vi "Convert LIN Trace to Raw Frame.vi"(8 "error in":errorcluster, 11 "captured data in":string[][](array[string])) -> (0 "error out":errorcluster, 2 "raw frames":u8[](array[numeric]) format="%02x")   [LabVIEW 2025, in "CAN-LIN Raw Bus Capture UI.lvlib"]
uses:
  CAN-LIN Raw Bus Capture UI.lvlib
  <vilib>/xnet/xnet.llb/XNET Frame Type LIN.ctl
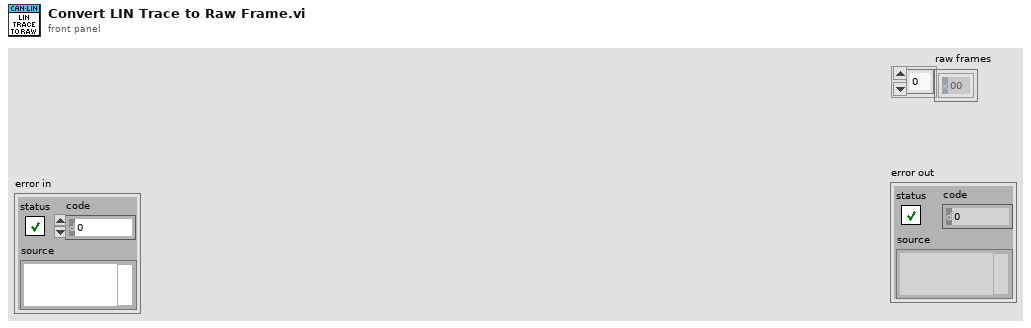
[diagram p1: front panel]
types:
  T1 = typedef "XNET Frame Type LIN.ctl" = u8
  T2 = cluster{"timestamp":timestamp, "payload":u8[], "identifier":u32, "type":T1, "event ID":u8, "event slot?":bool, "echo?":bool}[]
  T3 = cluster{"timestamp":timestamp, "payload":u8[], "identifier":u32, "type":T1, "event ID":u8, "event slot?":bool, "echo?":bool}
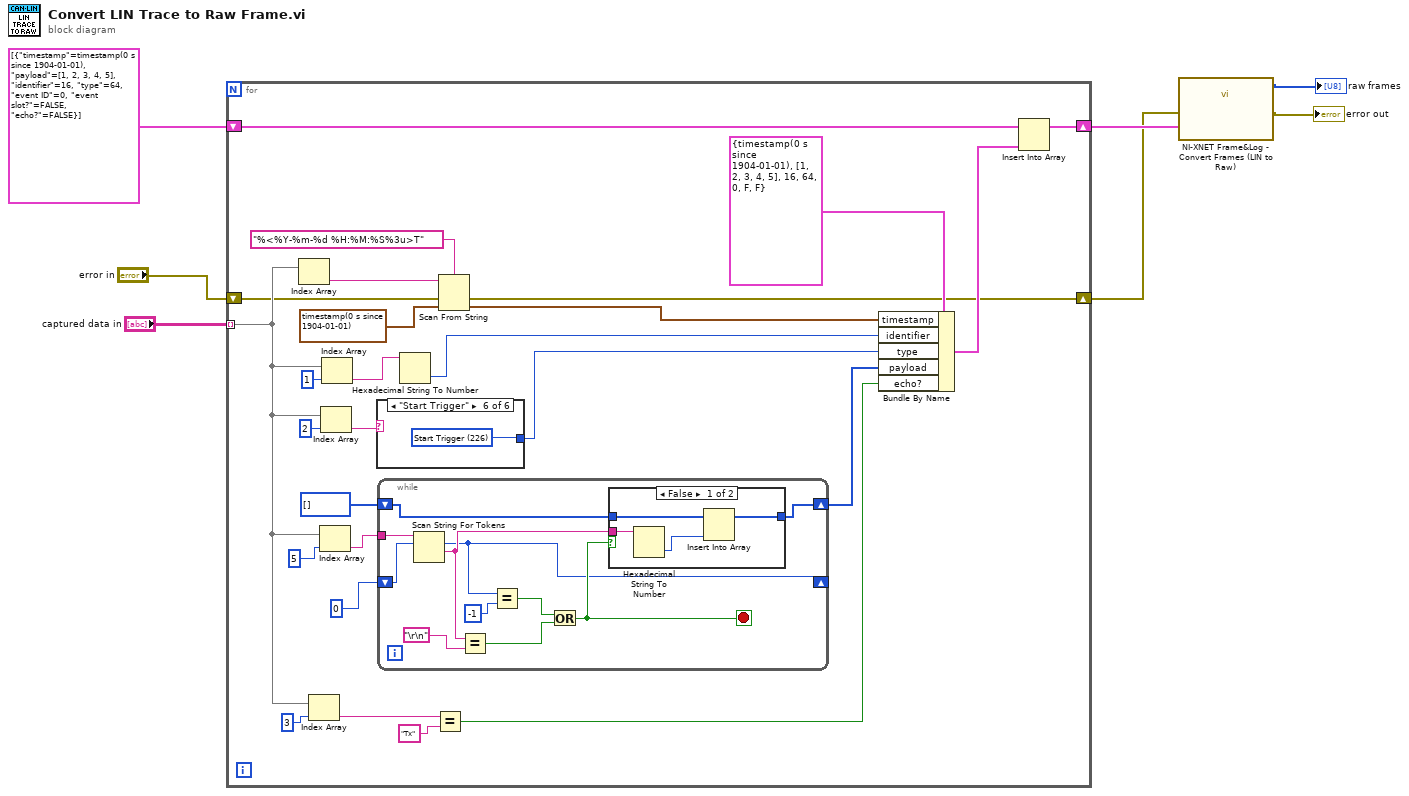
[diagram p0: block diagram]
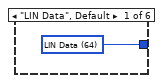
[diagram p3: hidden frame]
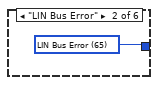
[diagram p4: hidden frame]
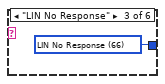
[diagram p5: hidden frame]
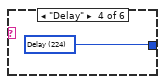
[diagram p6: hidden frame]
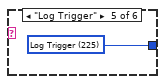
[diagram p7: hidden frame]
diagram:
  n1 = for {
    tunnel: "captured data in" -> [w16] mode=indexing
    shift-right: [w31] -> w5
    shift-left: T2 [{"timestamp"=timestamp(0 s since 1904-01-01), "payload"=[1, 2, 3, 4, 5], "identifier"=16, "type"=64, "event ID"=0, "event slot?"=FALSE, "echo?"=FALSE}] ("LIN frame") -> [w32]
    shift-right: [w9] -> w1
    shift-left: "error in" -> [w10]
    n2 = Index Array(array=w16) -> (element=w29:string)  [unwired: 1 in]
    n3 = Index Array(array=w16, index=3) -> (element=w14:string)
    n4 = Index Array(array=w16, index=5) -> (element=w20:string)
    n5 = Index Array(array=w16, index=2) -> (element=w23:string)
    n6 = Index Array(array=w16, index=1) -> (element=w26:string)
    n7 = case shown="\"Start Trigger\"" w23 {
      tunnel: [w50 w51 w52 w53 w54 w55] -> w22
      frame "LIN Data", Default {
        w50 = T1 64 items=["LIN Data"=64, "LIN Bus Error"=65, "LIN No Response"=66, "Delay"=224, "Log Trigger"=225, "Start Trigger"=226] ("type")
      }
      frame "LIN Bus Error" {
        w51 = T1 65 items=["LIN Data"=64, "LIN Bus Error"=65, "LIN No Response"=66, "Delay"=224, "Log Trigger"=225, "Start Trigger"=226] ("type")
      }
      frame "LIN No Response" {
        w52 = T1 66 items=["LIN Data"=64, "LIN Bus Error"=65, "LIN No Response"=66, "Delay"=224, "Log Trigger"=225, "Start Trigger"=226] ("type")
      }
      frame "Delay" {
        w53 = T1 224 items=["LIN Data"=64, "LIN Bus Error"=65, "LIN No Response"=66, "Delay"=224, "Log Trigger"=225, "Start Trigger"=226] ("type")
      }
      frame "Log Trigger" {
        w54 = T1 225 items=["LIN Data"=64, "LIN Bus Error"=65, "LIN No Response"=66, "Delay"=224, "Log Trigger"=225, "Start Trigger"=226] ("type")
      }
      frame "Start Trigger" {
        w55 = T1 226 items=["LIN Data"=64, "LIN Bus Error"=65, "LIN No Response"=66, "Delay"=224, "Log Trigger"=225, "Start Trigger"=226] ("type")
      }
    }
    n8 = while {
      tunnel: w20 -> [w44]
      shift-right: [w41] -> w18
      shift-left: u8[] [] ("payload") -> [w42]
      shift-right: [w34] -> _
      shift-left: 0 ("offset") -> [w39]
      stop <- w35 stop-if-true
      n9 = Scan String For Tokens(8:w39, 9:w44) -> (1:w40:string, 2:w34:i32)  [unwired: 4 in, 2 out]
      n10 = Equal?(x=w40, y="\r\n") -> (x = y?=w36:bool)
      n11 = Equal?(x=w34, y=-1) -> (x = y?=w37:bool)
      n12 = Or(x=w37, y=w36) -> (x .or. y?=w35:bool)
      n13 = case shown="False" w35 {
        tunnel: w42 -> [w47 w49]
        tunnel: [w45 w49] -> w41
        tunnel: w40 -> [w48 _]
        frame False {
          n14 = Hexadecimal String To Number(string=w48) -> (number=w46:u32)  [unwired: 2 in, 1 out]
          n15 = Insert Into Array(array=w47, new element=w46) -> (w45:u8[])  [unwired: 1 in]
        }
        frame True {
        }
      }
    }
    n16 = Hexadecimal String To Number(string=w26) -> (number=w25:u32)  [unwired: 2 in, 1 out]
    n17 = Equal?(x=w14, y="Tx") -> (x = y?=w12:bool)
    n18 = Scan From String(format string="%<%Y-%m-%d %H:%M:%S%3u>T", input string=w29, error in=w10, default 1=timestamp(0 s since 1904-01-01) ("timestamp")) -> (error out=w9:errorcluster, output 1=w28:timestamp)  [unwired: 1 in, 2 out]
    n19 = Bundle By Name(cluster=T3 {"timestamp"=timestamp(0 s since 1904-01-01), "payload"=[1, 2, 3, 4, 5], "identifier"=16, "type"=64, "event ID"=0, "event slot?"=FALSE, "echo?"=FALSE} ("LIN frame"), "timestamp"=w28, "identifier"=w25, "type"=w22, "payload"=w18, "echo?"=w12) -> (w33:T3)
    n20 = Insert Into Array(array=w32, new element=w33) -> (w31:T2)  [unwired: 1 in]
  }
  n21 = call "NI-XNET Frame&Log - Convert Frames (LIN to Raw).vi"("LIN frames"=w5, "error in"=w1) -> ("raw frames"=→"raw frames":u8[], "error out"=→"error out":errorcluster)  [unwired: 11 in, 1 out]
